vi "fahrenheit_celcius.vi"() -> ()   [LabVIEW 2019]
panel:
  out "concatenated string":string
  in  "stop":bool
  out "SICAKLIK":dbl
  out "Thermometer":dbl(slide) scale=0.0..200.0
  in  "SICAKLIK GİR":dbl
  in  "fahrenayt":bool
  # "Celcius"
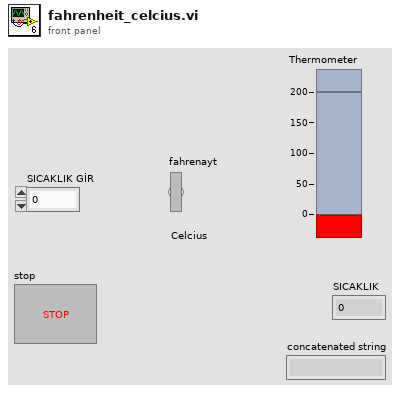
[diagram p1: front panel]
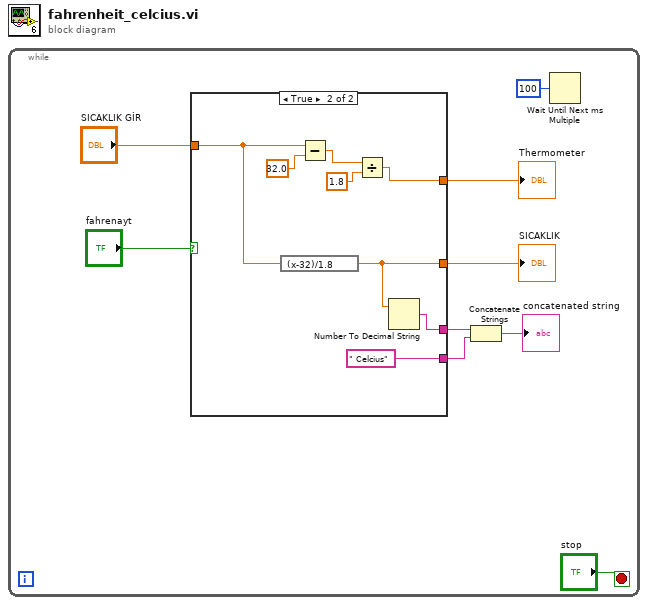
[diagram p0: block diagram]
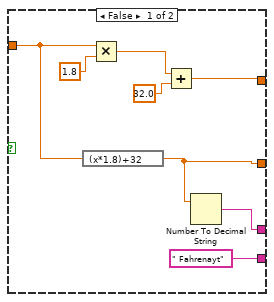
[diagram p2: hidden frame]
diagram:
  n1 = while {
    stop <- "stop" stop-if-true
    n2 = case shown="True" "fahrenayt" {
      tunnel: "SICAKLIK GİR" -> [w10 w21]
      tunnel: [w14 w22] -> w5
      tunnel: [w15 w19] -> w4
      tunnel: [" Fahrenayt" ("string") " Celcius" ("string")] -> w2
      tunnel: [w16 w18] -> w1
      frame False {
        n3 = expression code="(x*1.8)+32"(w10) -> (w15:dbl)
        n4 = Multiply(x=w10, y=1.8) -> (x*y=w12:dbl)
        n5 = Add(x=w12, y=32.0) -> (x+y=w14:dbl)
        n6 = Number To Decimal String(number=w15) -> (decimal integer string=w16:string)  [unwired: 1 in]
      }
      frame True {
        n7 = expression code="(x-32)/1.8"(w21) -> (w19:dbl)
        n8 = Subtract(x=w21, y=32.0) -> (x-y=w23:dbl)
        n9 = Divide(x=w23, y=1.8) -> (x/y=w22:dbl)
        n10 = Number To Decimal String(number=w19) -> (decimal integer string=w18:string)  [unwired: 1 in]
      }
    }
    "Thermometer" <- w5
    "SICAKLIK" <- w4
    n11 = Concatenate Strings(w1, w2) -> (→"concatenated string":string)
    n12 = Wait Until Next ms Multiple(millisecond multiple=u32 100) -> ()  [unwired: 1 out]
  }
